vi "Load Zplane_Pockels_Values dat file.vi"(11 "Experiment data folder path":path) -> (0 "[AOL Z (um)]":dbl[](array[numeric]), 1 "Zplane_Pockels_Values file data (header removed)":dbl[][](array[numeric]), 2 "2D array size":i32[](array[numeric]), 3 "Columns header":string[](array[string]), 4 "Zplane Pockels values file exists":bool, 5 "Version index (-1 = latest version)":i32)   [LabVIEW 2020]
uses:
  Typedefs/Enum-Which file or folder.ctl
  <userlib>/My Palettes.lib/Files & paths/Spreadsheet/Read From Spreadsheet File (string)-Mod.vi
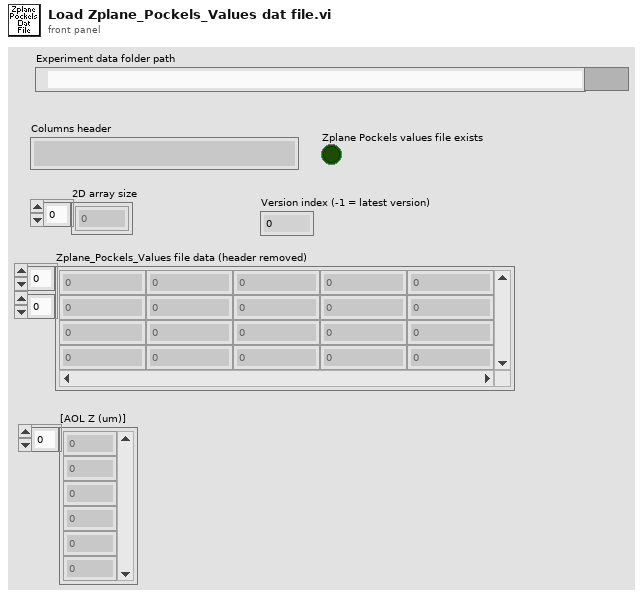
[diagram p1: front panel]
types:
  T1 = typedef "Enum-Which file or folder.ctl" = enum16{"ROI file", "Normalised ROI file", "Zplane Pockels values file", "Functional data folder"}
  T2 = typedef "Fixed strings.ctl" = cluster{"ROI file name":string, "Normalised ROI file name":string, "Zplane Pockels values file name":string, "Functional data folder name":string, "Experiment Header file name":string, "Z-stack images folder name":string, "Groups setup rel. path":string, "Groups text file rel. path":string, "TDMS files folder name (F.img)":string, "TDMS files folder name (V.acq)":string, "TDMS files folder name (Pl.acq)":string, "Cycle rel times sequence file":string, "Dynamically called VIs folder name":string, "Time Series folder base name":string}
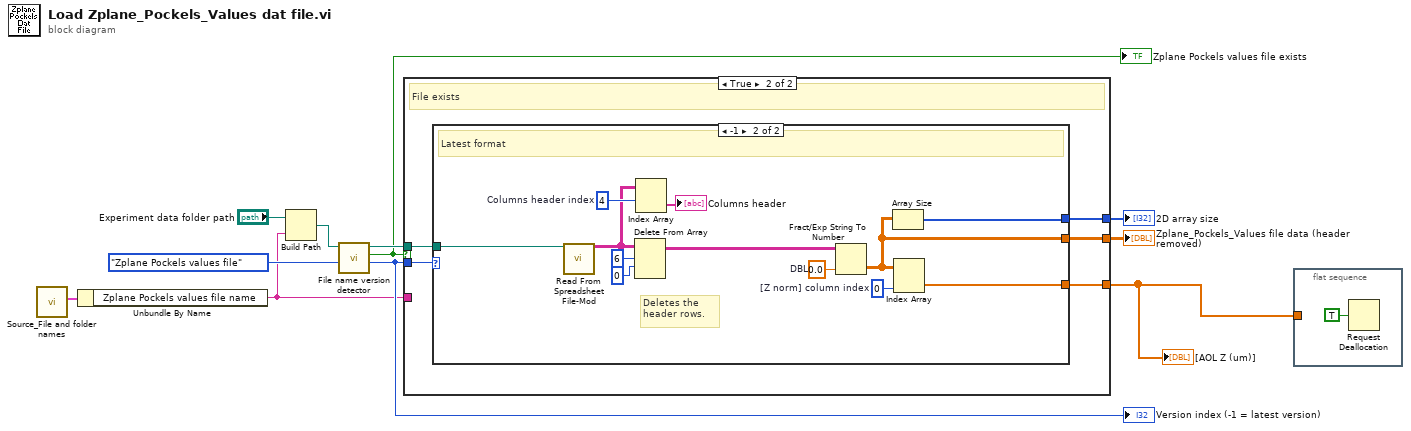
[diagram p0: block diagram]
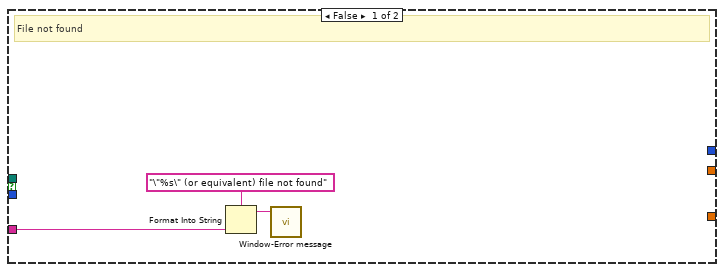
[diagram p2: hidden frame]
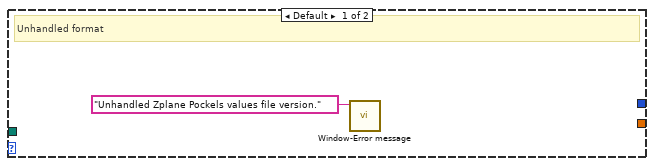
[diagram p3: hidden frame]
diagram:
  n1 = call "Source_File and folder names.vi"() -> ("Fixed strings"=w2:T2)  [unwired: 1 in]
  n2 = Unbundle By Name(w2) -> ("Zplane Pockels values file name"=w3:string)
  n3 = Build Path(base path="Experiment data folder path", name or relative path=w3) -> (appended path=w7:path)
  n4 = call "File name version detector.vi"("Which file/folder?"=Enum-Which_file_or_folder."Zplane Pockels values file", "Path in"=w7) -> ("Version index (-1 = latest version)"=w5:i32, "file or folder exists"=w4:bool, "Path out"=w6:path)  [unwired: 7 in]
  "Version index (-1 = latest version)" <- w5
  "Zplane Pockels values file exists" <- w4
  n5 = case shown="True" w4 {
    tunnel: [_ w19] -> w11
    tunnel: [_ w18] -> w10
    tunnel: [_ w17] -> w1
    tunnel: w6 -> [_ w16]
    tunnel: w3 -> [w13 _]
    tunnel: w5 -> [_ w15]
    frame False {
      # "File not found"
      n6 = Format Into String(format string="\"%s\" (or equivalent) file not found" ("message"), w13) -> (resulting string=w12:string)  [unwired: 2 in, 1 out]
      n7 = call "Window-Error message.vi"("Message"=w12) -> ()  [unwired: 10 in, 1 out]
    }
    frame True {
      # "File exists"
      n8 = case shown="-1" w15 {
        tunnel: [_ w29] -> w19
        tunnel: [_ w28] -> w18
        tunnel: [_ w27] -> w17
        tunnel: w16 -> [_ w22]
        frame Default {
          # "Unhandled format"
          n9 = call "Window-Error message.vi"("Message"="Unhandled Zplane Pockels values file version." ("message")) -> ()  [unwired: 10 in, 1 out]
        }
        frame -1 {
          w32 = 4  # Columns header index
          w30 = 0.0  # DBL
          w26 = 0  # [Z norm] column index
          # "Deletes the header rows."
          # "Latest format"
          n10 = call-poly <userlib>:"Read From Spreadsheet File-Mod.vi"("file path (dialog if empty)"=w22) -> ("all rows"=w21:string[][])  [unwired: 9 in, 5 out]
          n11 = Delete From Array "Delete From Array"(array=w21, length=6, index (row)=0) -> (array with subset deleted=w25:string[][])  [unwired: 1 in, 1 out]
          n12 = Index Array(array=w21, index (row)=w32) -> (element=→"Columns header":string[])  [unwired: 1 in]
          n13 = Fract/Exp String To Number(string=w25, default (0 dbl)=w30) -> (number=w29:dbl[][])  [unwired: 2 in, 1 out]
          n14 = Array Size(array=w29) -> (size(s)=w28:i32[])
          n15 = Index Array(array=w29, index (col)=w26) -> (element=w27:dbl[])  [unwired: 1 in]
        }
      }
    }
  }
  "Zplane_Pockels_Values file data (header removed)" <- w11
  "2D array size" <- w10
  "[AOL Z (um)]" <- w1
  n16 = flat-sequence {
    tunnel: w1 -> [_]
    frame #0 {
      n17 = Request Deallocation(TRUE ("flag")) -> ()
    }
  }
